vi "Part-23-LabVIEW-Sound.vi"() -> ()   [LabVIEW 2015]
uses:
  <userlib>/TripleDisplayX.llb/TripleDisplay.xctl
panel:
  in  "sampling info":cluster{"Fs":dbl, "#s":dbl}={"Fs"=1000.0, "#s"=1000.0} {"Fs" format="%.2p"}
  in  "signal type":T1(ring)
  in  "phase":dbl format="%.2p"
  in  "amplitude":dbl=1.0 format="%0.2p"
  in  "frequency":dbl=10.0 format="%0.2p"
  out "TripleDisplay":waveform(dbl)(xcontrol)
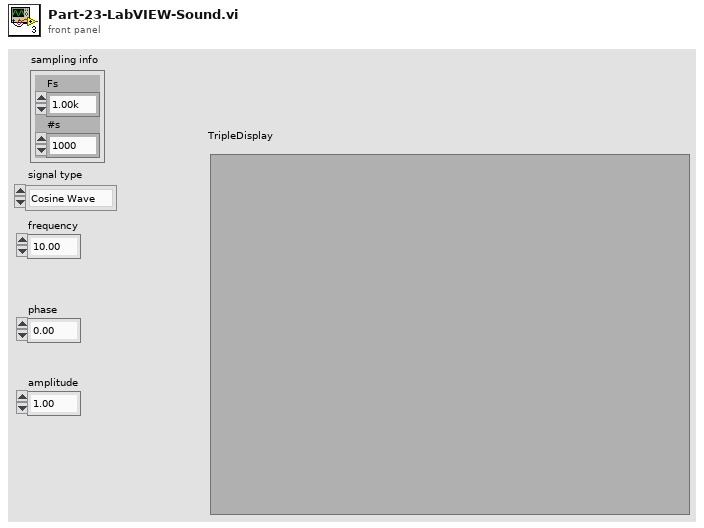
[diagram p1: front panel]
types:
  T1 = enum16{"Cosine Wave", "Sine Wave", "Triangle Wave", "Square Wave", "Sawtooth Wave"}
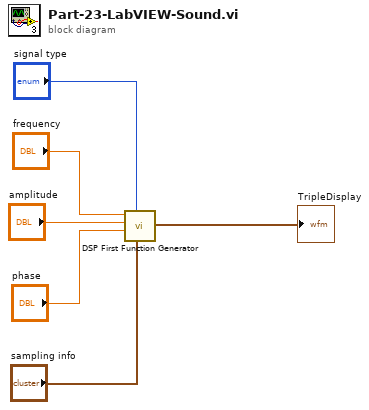
[diagram p0: block diagram]
diagram:
  n1 = call <userlib>:"DSP First Function Generator.vi"("sampling info"="sampling info", "signal type"="signal type", "phase"="phase", "amplitude"="amplitude", "frequency"="frequency") -> ("signal out"=→"TripleDisplay":waveform(dbl))  [unwired: 4 in, 2 out]
